vi "Custom VI Periodic IO Server.vi"() -> ()   [LabVIEW 2021]
panel:
  in  "Iteration Rate":u32=200
  out "Heater":bool
  in  "stop":bool
  out "Thermometer":dbl(slide) scale=0.0..100.0
  out "Waveform Chart":dynamicdata(graph)
  in  "Lower Temp. Set Point":i32(knob)=40 scale=40.0..60.0
  in  "Max. Temp. Set Point":i32(knob)=70 scale=60.0..80.0
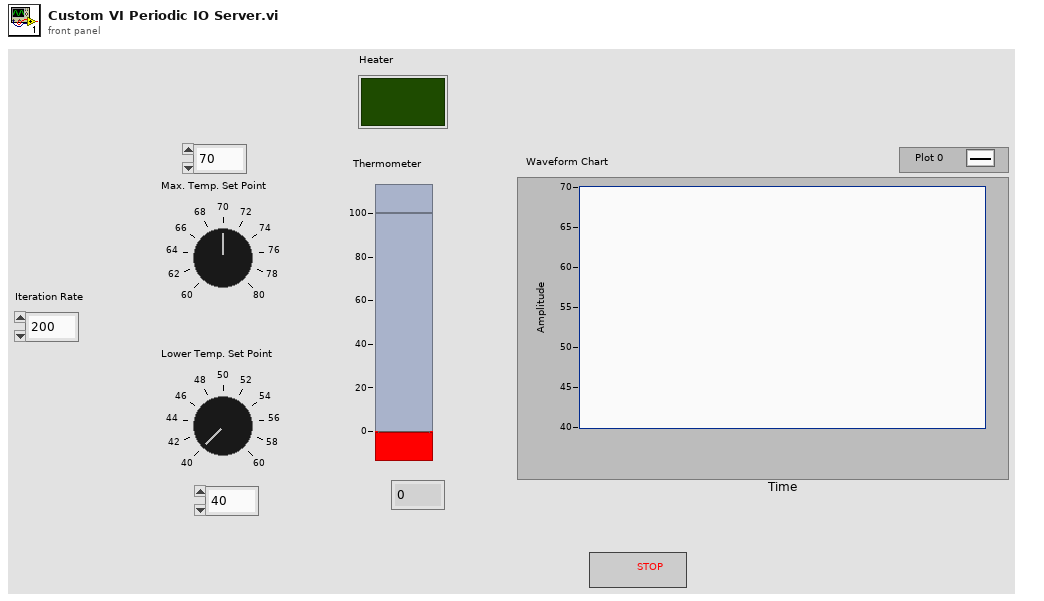
[diagram p1: front panel]
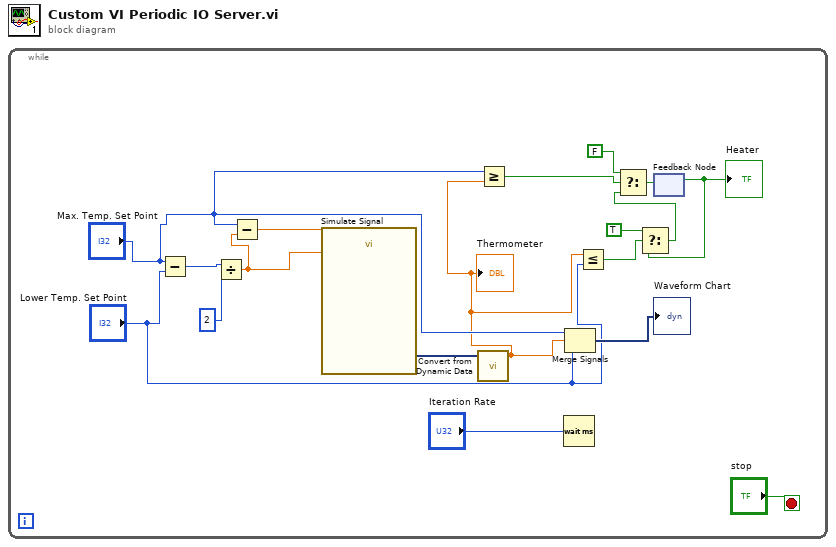
[diagram p0: block diagram]
diagram:
  n1 = while {
    stop <- "stop" stop-if-true
    n2 = Subtract(x="Max. Temp. Set Point", y="Lower Temp. Set Point") -> (x-y=w18:i32)
    n3 = Divide(x=w18, y=2) -> (x/y=w16:dbl)
    n4 = Subtract(x="Max. Temp. Set Point", y=w16) -> (x-y=w15:dbl)
    n5 = call "Simulate Signal"("Offset"=w15, "Amplitude"=w16) -> ("Sine with Uniform Noise"=w14:dynamicdata)  [unwired: 12 in, 1 out]
    n6 = call "Convert from Dynamic Data"("Dynamic Data Type"=w14) -> ("Scalar"=w9:dbl)  [unwired: 3 in]
    "Thermometer" <- w9
    n7 = Greater Or Equal?(x="Max. Temp. Set Point", y=w9) -> (x >= y?=w8:bool)
    n8 = Wait (ms)(milliseconds to wait="Iteration Rate") -> ()  [unwired: 1 out]
    n9 = Merge Signals("Max. Temp. Set Point", w9, "Lower Temp. Set Point") -> (→"Waveform Chart":dynamicdata)
    n10 = Less Or Equal?(x=w9, y="Lower Temp. Set Point") -> (x <= y?=w7:bool)
    n11 = feedback #1() -> (w2:bool)  [unwired: 1 in]
    "Heater" <- w2
    n12 = Select(t=TRUE, s=w7, f=w2) -> (s? t:f=w4:bool)
    n13 = Select(t=FALSE, s=w8, f=w4) -> (s? t:f=w3:bool)
    n14 = feedback-in #1(w3) -> ()
  }
